vi "Compare_Values_Assign_Costs-1.vi"(4 "[IN] Array of displa\ncement differences":dbl[](array[numeric]), 5 "[IN] Cost function":i8[](array[numeric]), 6 "[IN] Track Length":u8[](array[numeric]), 7 "[IN] Array of displacements":dbl[](array[numeric]), 8 "[IN] Statuses of points":i16[](array[numeric]), 9 "[IN] Areas \ndifferences":dbl[](array[numeric]), 10 "[IN] Reverse or not":bool[](array[boolean]), 11 "[IN] Angles betwe\nen displacements":dbl[](array[numeric])) -> (3 "[OUT] Cost function":i8[](array[numeric]))   [LabVIEW 2013]
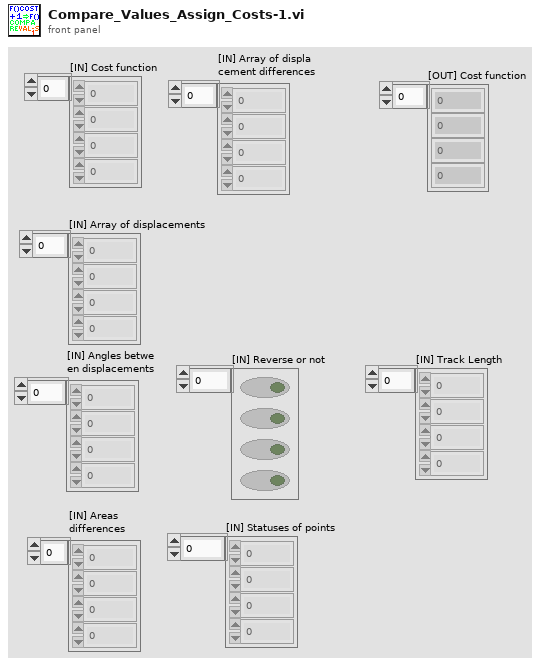
[diagram p1: front panel]
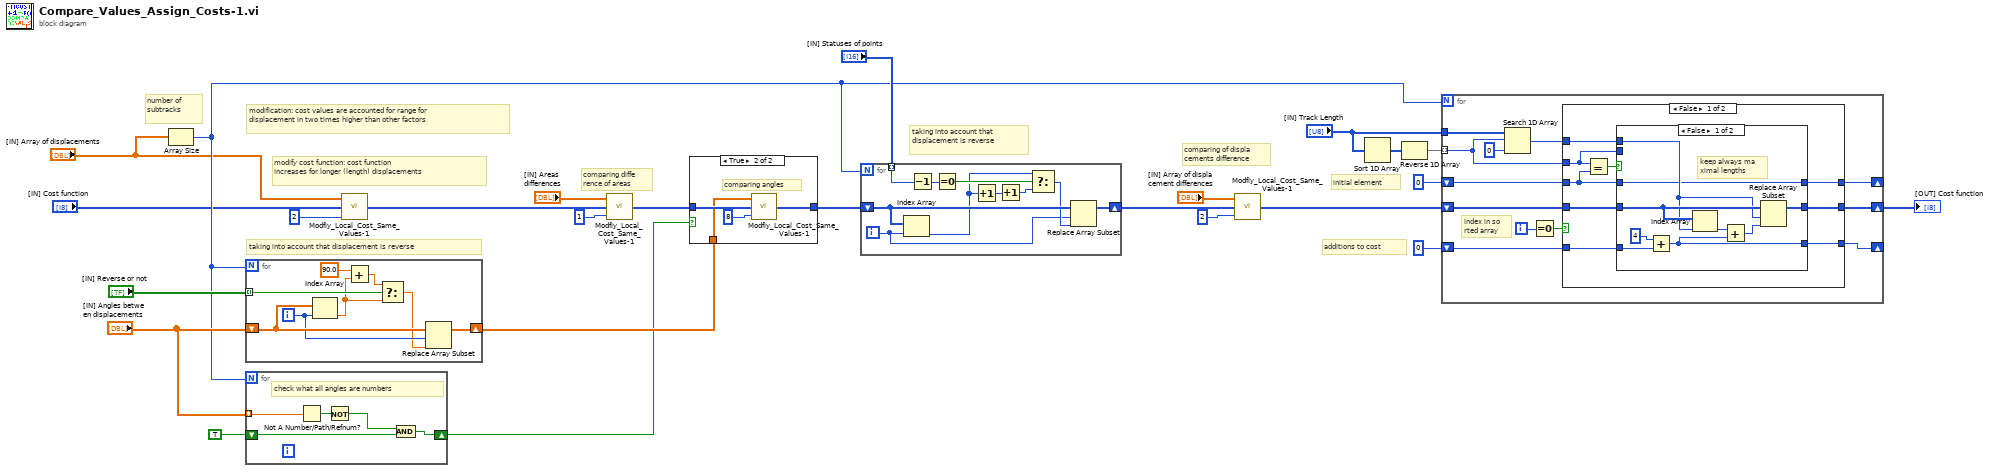
[diagram p0: block diagram]
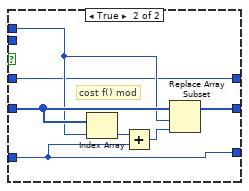
[diagram p3: hidden frame]
diagram:
  # "comparing of displa\ncements difference"
  # "comparing diffe\nrence of areas"
  # "modification: cost values are accounted for range for \ndisplacement in two times higher than other factors"
  # "additions to cost"
  # "initial element"
  # "taking into account that \ndisplacement is reverse"
  # "taking into account that displacement is reverse"
  # "modify cost function: cost function \nincreases for longer (length) displacements"
  # "number of \nsubtracks"
  n1 = Array Size(array="[IN] Array of displacements") -> (size(s)=w12:i32)
  n2 = for {
    N: w12 -> [_]
    tunnel: "[IN] Angles betwe\nen displacements" -> [w29] mode=indexing
    shift-right: [w26] -> w13
    shift-left: TRUE -> [w30]
    # "check what all angles are numbers"
    n3 = Not A Number/Path/Refnum?(number/path/refnum=w29) -> (NaN/Path/Refnum?=w28:bool)
    n4 = Not(x=w28) -> (.not. x?=w27:bool)
    n5 = And(x=w27, y=w30) -> (x .and. y?=w26:bool)
  }
  n6 = for {
    N: w12 -> [_]
    shift-right: [w31] -> w24
    shift-left: "[IN] Angles betwe\nen displacements" -> [w37]
    tunnel: "[IN] Reverse or not" -> [w38] mode=indexing
    i -> [w33]
    n7 = Index Array(array=w37, index=w33) -> (element=w35:dbl)
    n8 = Add(x=90.0, y=w35) -> (x+y=w34:dbl)
    n9 = Select(t=w34, s=w38, f=w35) -> (s? t:f=w32:dbl)
    n10 = Replace Array Subset(array=w37, new element=w32, index=w33) -> (w31:dbl[])
  }
  n11 = call "Modfiy_Local_Cost_Same_Values-1.vi"("[IN] Cost Mutilplier"=i8 2, "[IN] Cost Function"="[IN] Cost function", "[IN] Array of Compared Values"="[IN] Array of displacements") -> ("[OUT] Cost Function"=w8:i8[])  [unwired: 2 in]
  n12 = call "Modfiy_Local_Cost_Same_Values-1.vi"("[IN] Cost Mutilplier"=i8 1, "[IN] Cost Function"=w8, "[IN] Array of Compared Values"="[IN] Areas \ndifferences") -> ("[OUT] Cost Function"=w5:i8[])  [unwired: 2 in]
  n13 = case shown="True" w13 {
    tunnel: w24 -> [_ w42]
    tunnel: w5 -> [w39 w43]
    tunnel: [w39 w40] -> w23
    frame False {
    }
    frame True {
      # "comparing angles"
      n14 = call "Modfiy_Local_Cost_Same_Values-1.vi"("[IN] Cost Mutilplier"=i8 8, "[IN] Cost Function"=w43, "[IN] Array of Compared Values"=w42) -> ("[OUT] Cost Function"=w40:i8[])  [unwired: 2 in]
    }
  }
  n15 = for {
    N: w12 -> [_]
    shift-right: [w44] -> w4
    shift-left: w23 -> [w53]
    tunnel: "[IN] Statuses of points" -> [w52] mode=indexing
    i -> [w45]
    n16 = Index Array(array=w53, index=w45) -> (element=w49:i8)
    n17 = Decrement(x=w52) -> (x-1=w51:i16)
    n18 = Equal To 0?(x=w51) -> (x = 0?=w50:bool)
    n19 = Increment(x=w49) -> (x+1=w48:i8)
    n20 = Increment(x=w48) -> (x+1=w47:i8)
    n21 = Select(t=w49, s=w50, f=w47) -> (s? t:f=w46:i8)
    n22 = Replace Array Subset(array=w53, new element=w46, index=w45) -> (w44:i8[])
  }
  n23 = call "Modfiy_Local_Cost_Same_Values-1.vi"("[IN] Cost Mutilplier"=i8 2, "[IN] Cost Function"=w4, "[IN] Array of Compared Values"="[IN] Array of displa\ncement differences") -> ("[OUT] Cost Function"=w2:i8[])  [unwired: 2 in]
  n24 = Sort 1D Array(array="[IN] Track Length") -> (sorted array=w21:u8[])
  n25 = Reverse 1D Array(array=w21) -> (reversed array=w20:u8[])
  n26 = for {
    N: w12 -> [_]
    tunnel: w20 -> [w61] mode=indexing
    tunnel: "[IN] Track Length" -> [w65]
    shift-right: [w59] -> w16
    shift-left: w2 -> [w60]
    shift-right: [w58] -> _
    shift-left: u8 0 -> [w57]
    shift-right: [w55] -> _
    shift-left: i8 0 -> [w56]
    i -> [w63]
    # "index in so\nrted array"
    n27 = Search 1D Array(1D array=w65, element=w61, start index (0)=0) -> (index of element=w54:i32)
    n28 = Equal To 0?(x=w63) -> (x = 0?=w62:bool)
    n29 = case shown="False" w62 {
      tunnel: w61 -> [w70 w92]
      tunnel: [w69 w93] -> w59
      tunnel: w60 -> [w73 w93]
      tunnel: [w68 w92] -> w58
      tunnel: w57 -> [w66 _]
      tunnel: [w67 w91] -> w55
      tunnel: w56 -> [w71 w91]
      tunnel: w54 -> [w72 _]
      frame False {
        n30 = Equal?(x=w70, y=w66) -> (x = y?=w74:bool)
        n31 = case shown="False" w74 {
          tunnel: w73 -> [w81 w88]
          tunnel: w72 -> [w78 w85]
          tunnel: w71 -> [w83 w87]
          tunnel: w70 -> [_ _]
          tunnel: [w77 w86] -> w69
          tunnel: [w75 w84] -> w68
          tunnel: [w76 w87] -> w67
          tunnel: w66 -> [w75 w84]
          frame False {
            # "keep always ma\nximal lengths"
            n32 = Add(x=i8 4 ("y"), y=w83) -> (x+y=w76:i8)
            n33 = Index Array(array=w81, index=w78) -> (element=w80:i8)
            n34 = Add(x=w80, y=w76) -> (x+y=w79:i8)
            n35 = Replace Array Subset(array=w81, new element=w79, index=w78) -> (w77:i8[])
          }
          frame True {
            # "cost f() mod"
            n36 = Index Array(array=w88, index=w85) -> (element=w89:i8)
            n37 = Add(x=w89, y=w87) -> (x+y=w90:i8)
            n38 = Replace Array Subset(array=w88, new element=w90, index=w85) -> (w86:i8[])
          }
        }
      }
      frame True {
        # "keep maximal length\nfor comparisons"
      }
    }
  }
  "[OUT] Cost function" <- w16
